vi "Dependency Info.vi"(8 "error in (no error)":errorcluster, 10 "From Folder":path, 11 "Package in":refnum<class "Package.lvclass">) -> (0 "error out":errorcluster, 2 "Dependency":T1)   [LabVIEW 2020, in "GPack.lvlib" / "Package.lvclass"]
uses:
  Package.lvclass
  Dependency.ctl
  Package Info.ctl
  GPack.lvlib
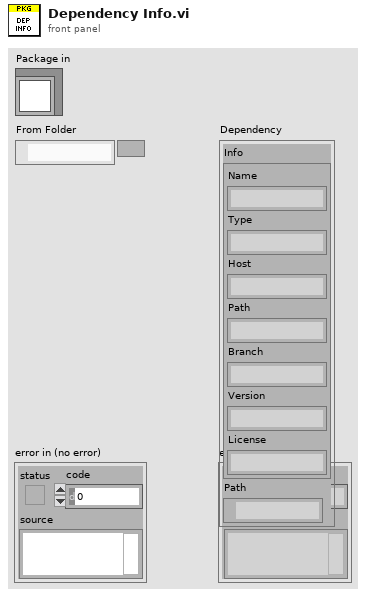
[diagram p1: front panel]
types:
  T1 = typedef "GPack.lvlib/Dependency.ctl" = cluster{"Info":T2, "Path":path}
  T2 = typedef "GPack.lvlib/Package Info.ctl" = cluster{"Name":string, "Type":string, "Host":string, "Path":string, "Branch":string, "Version":string, "License":string}
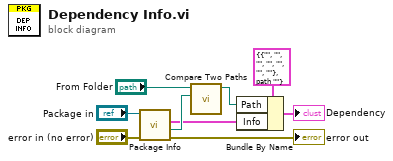
[diagram p0: block diagram]
diagram:
  n1 = call-dynamic "Package Info.vi"("error in (no error)"="error in (no error)", "Package in"="Package in") -> ("error out"=→"error out":errorcluster, "Folder"=w6:path, "Package Info"=w4:T2)  [unwired: 7 in]
  n2 = call <vilib>:"Compare Two Paths.vi"("Path 2"=w6, "Path 1"="From Folder") -> ("Relative Path from 1 to 2"=w3:path)  [unwired: 6 in, 3 out]
  n3 = Bundle By Name(cluster=T1 {"Info"={"Name"="", "Type"="", "Host"="", "Path"="", "Branch"="", "Version"="", "License"=""}, "Path"=path ""} ("Dependency"), "Path"=w3, "Info"=w4) -> (→"Dependency":T1)
